vi "GetRoots.vi"(11 "TreeControl in":refnum<vi>) -> (2 "Root Elements":cluster{"String":string, "Value":string}[](array[cluster]))   [LabVIEW 2014]
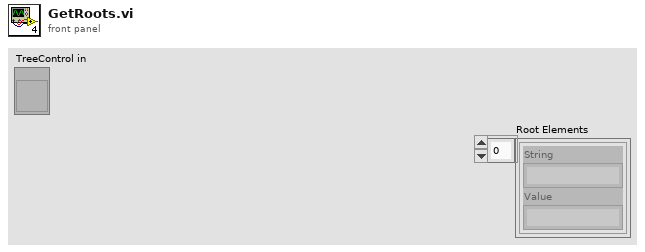
[diagram p1: front panel]
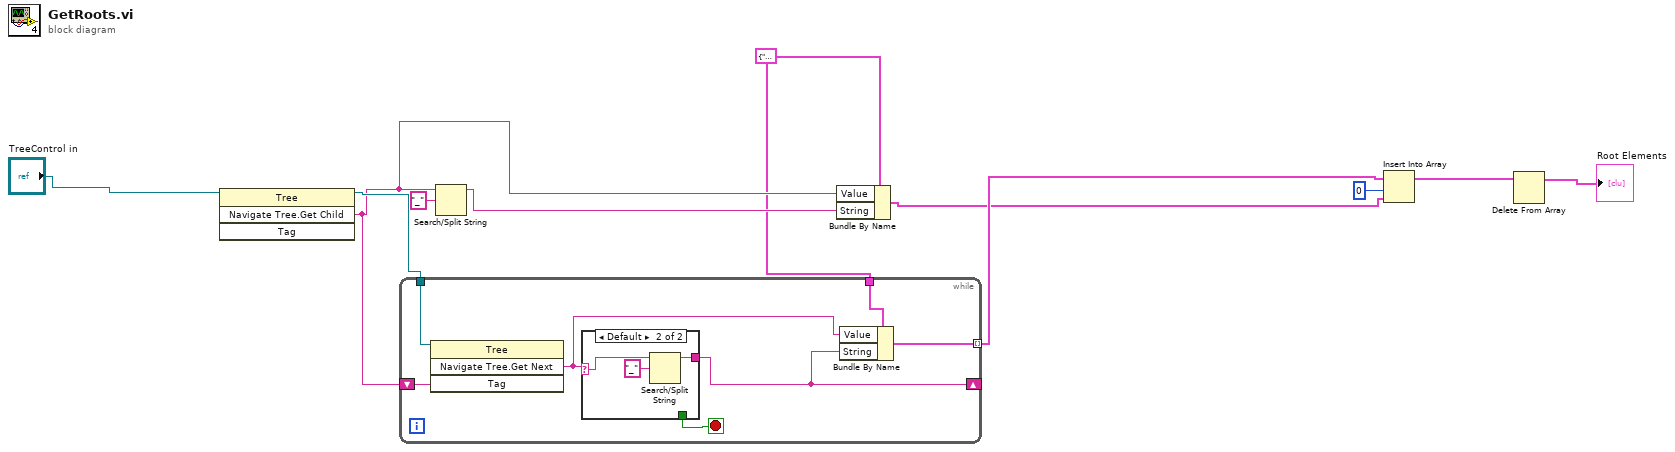
[diagram p0: block diagram]
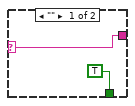
[diagram p2: hidden frame]
diagram:
  w3 = cluster{"String":string, "Value":string} {"String"="", "Value"=""}
  n1 = invoke class="Tree" method="Navigate Tree.Get Child"(reference="TreeControl in") -> (reference out=w11:refnum<vi>, "Navigate Tree:Get Child"=w6:string)  [unwired: 3 in, 2 out]
  n2 = while {
    tunnel: w11 -> [w16]
    shift-right: [w12] -> _
    shift-left: w6 -> [w18]
    tunnel: w3 -> [w15]
    tunnel: [w13] -> w7 mode=indexing
    stop <- w17 stop-if-true
    n3 = invoke class="Tree" method="Navigate Tree.Get Next"(reference=w16, "Tag"=w18) -> ("Navigate Tree:Get Next Item"=w14:string)  [unwired: 2 in, 3 out]
    n4 = case shown="Default" w14 {
      selector: w14 -> [w19 w23]
      tunnel: [w19 w21] -> w12
      tunnel: [TRUE _] -> w17
      frame "" {
      }
      frame Default {
        n5 = Search/Split String(string=w23, search string/char (-)="_") -> (substring before match=w21:string)  [unwired: 1 in, 2 out]
      }
    }
    n6 = Bundle By Name(cluster=w15, "Value"=w14, "String"=w12) -> (w13:cluster{"String":string, "Value":string})
  }
  n7 = Search/Split String(string=w6, search string/char (-)="_") -> (substring before match=w5:string)  [unwired: 1 in, 2 out]
  n8 = Bundle By Name(cluster=w3, "Value"=w6, "String"=w5) -> (w4:cluster{"String":string, "Value":string})
  n9 = Insert Into Array(array=w7, index=0, new element=w4) -> (w8:cluster{"String":string, "Value":string}[])
  n10 = Delete From Array(array=w8) -> (array with subset deleted=→"Root Elements":cluster{"String":string, "Value":string}[])  [unwired: 2 in, 1 out]
